vi "BinaryToFloatScaleFactor.vi"() -> (0 "Scale Factor":dbl)   [LabVIEW 2014]
doc: "Generates the Scale Factor to convert the Binary left justified (Most significant bit) 12-bit data stored in a 16-bit int to floating point.\nADC Voltage Resolution = Voltage Range / (ADC intervals *16)"
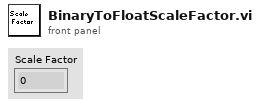
[diagram p1: front panel]
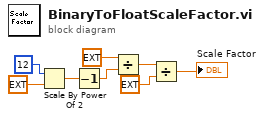
[diagram p0: block diagram]
diagram:
  n1 = Scale By Power Of 2(n=12, x=ext 1.0) -> (x*2^n=w4:ext)
  n2 = Decrement(x=w4) -> (x-1=w5:ext)
  n3 = Divide(x=ext 2.0, y=w5) -> (x/y=w7:ext)
  n4 = Divide(x=w7, y=ext 16.0) -> (x/y=→"Scale Factor":ext)
